vi "Finalize.vi"(8 "error in":errorcluster, 11 "Plugin in":refnum<class "Performanced XNET CAN Signal Logger.lvclass">) -> (0 "error out":errorcluster, 3 "Plugin out":refnum<class "Performanced XNET CAN Signal Logger.lvclass">)   [LabVIEW 2021, in "Performanced XNET CAN Signal Logger.lvlib" / "Performanced XNET CAN Signal Logger.lvclass"]
uses:
  Performanced XNET CAN Signal Logger.lvclass
  Typedef/Def-Executor Command.ctl
  Performanced XNET CAN Signal Logger.lvclass/Performanced XNET CAN Signal Logger.ctl
  XNET-CAN-Signal-Logger.lvlib
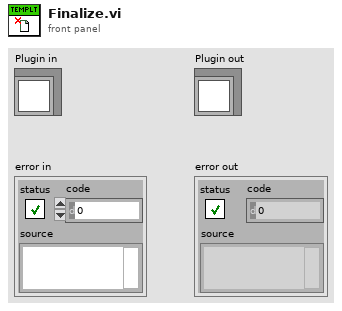
[diagram p1: front panel]
types:
  T1 = typedef "XNET-CAN-Signal-Logger.lvlib/Def-Executor Command.ctl" = cluster{"Command":string, "Data":variant}
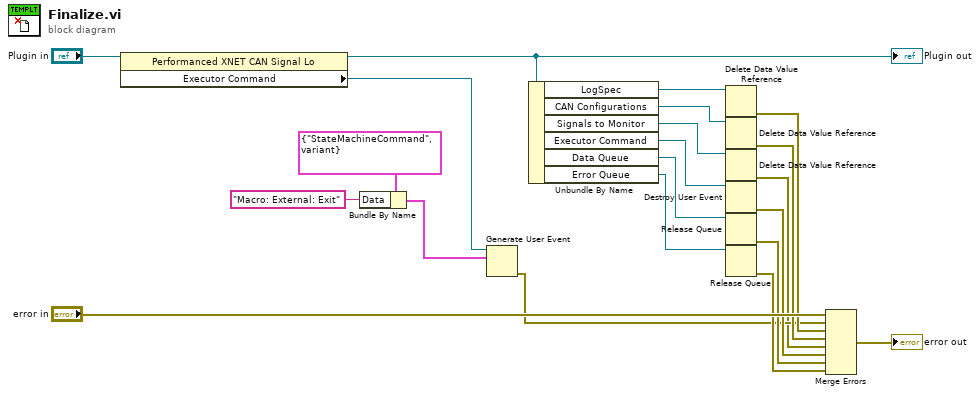
[diagram p0: block diagram]
diagram:
  n1 = property class="Performanced XNET CAN Signal Lo"(reference="Plugin in") -> (reference out=w7:refnum<class "Performanced XNET CAN Signal Logger.lvclass">, "Executor Command"=w3:refnum<user-event>)  [unwired: 1 in, 1 out]
  "Plugin out" <- w7
  n2 = Bundle By Name(cluster=T1 {"Command"="StateMachineCommand", "Data"=variant} ("event data"), "Data"="Macro: External: Exit") -> (w5:T1)
  n3 = Generate User Event(user event=w3, event data cluster=w5) -> (error out=w2:errorcluster)  [unwired: 2 in, 1 out]
  n4 = Unbundle By Name(w7) -> ("LogSpec"=w16:refnum<data-value>, "CAN Configurations"=w15:refnum<data-value>, "Signals to Monitor"=w14:refnum<data-value>, "Executor Command"=w13:refnum<user-event>, "Data Queue"=w11:refnum<queue>, "Error Queue"=w12:refnum<queue>)
  n5 = Delete Data Value Reference(data value reference=w16) -> (error out=w19:errorcluster)  [unwired: 1 in, 1 out]
  n6 = Delete Data Value Reference(data value reference=w15) -> (error out=w18:errorcluster)  [unwired: 1 in, 1 out]
  n7 = Delete Data Value Reference(data value reference=w14) -> (error out=w1:errorcluster)  [unwired: 1 in, 1 out]
  n8 = Destroy User Event(user event=w13) -> (error out=w8:errorcluster)  [unwired: 1 in]
  n9 = Release Queue(queue=w11) -> (error out=w9:errorcluster)  [unwired: 2 in, 2 out]
  n10 = Release Queue(queue=w12) -> (error out=w10:errorcluster)  [unwired: 2 in, 2 out]
  n11 = Merge Errors("error in", w2, w19, w18, w1, w8, w9, w10) -> (→"error out":errorcluster)
